vi "ForceSelect.vi"(9 "Input Function":i32 min=0 max=2 step=1) -> (1 "Force Function":string)   [LabVIEW 2023]
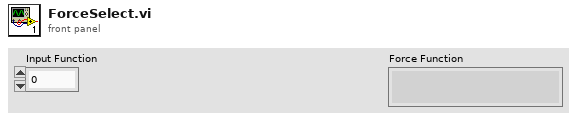
[diagram p1: front panel]
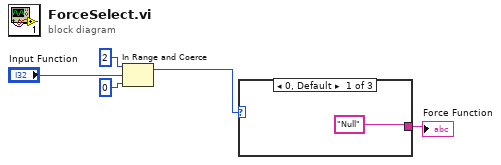
[diagram p0: block diagram]
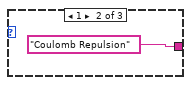
[diagram p2: hidden frame]
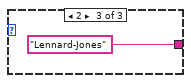
[diagram p3: hidden frame]
diagram:
  n1 = In Range and Coerce(upper limit=2, x="Input Function", lower limit=0) -> (coerced(x)=w1:i32)  [unwired: 1 out]
  n2 = case shown="0, Default" w1 {
    tunnel: ["Null" "Coulomb Repulsion" "Lennard-Jones"] -> w2
    frame 0, Default {
    }
    frame 1 {
    }
    frame 2 {
    }
  }
  "Force Function" <- w2
